vi "Color Pixel with Color Scale.vi"(6 "Color Scale 1D Color Array":T2(array[cluster]), 7 "Limit+NaN Colors":T1, 8 "Error In":errorcluster, 9 "Color Scale Min Value":sgl, 10 "Color Scale Max Value":sgl, 11 "Pixel Value":sgl) -> (0 "Error Out":errorcluster, 3 "Pixel Color":T3)   [LabVIEW 2021, in "Image.lvlib"]
uses:
  Palette/Limit+NaN Colors.ctl
  Image.lvlib
  Palette/Palette.lvlib
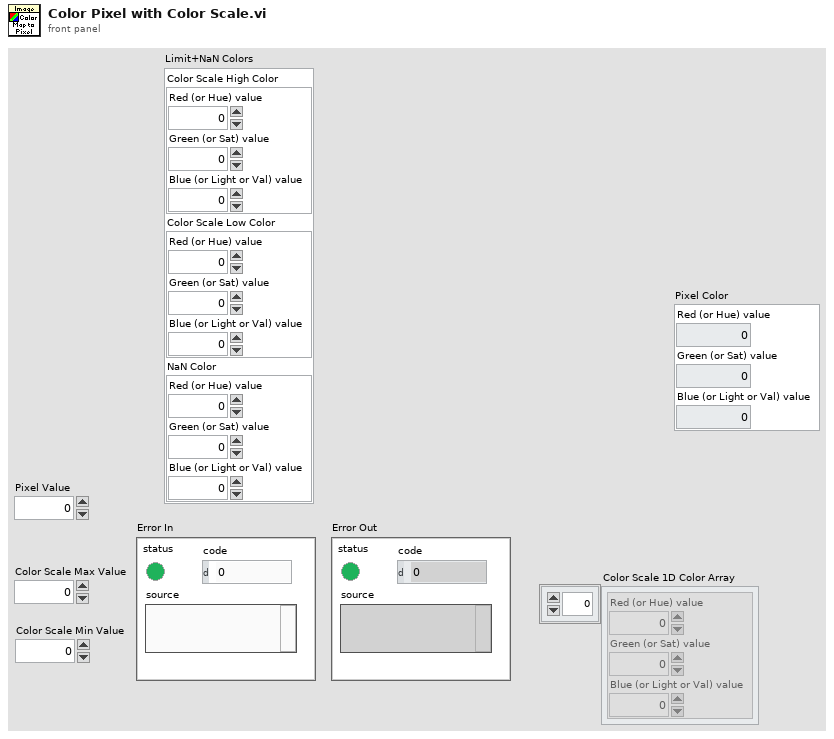
[diagram p1: front panel]
types:
  T1 = typedef "Palette.lvlib/Limit+NaN Colors.ctl" = cluster{"Color Scale High Color":cluster{"Red (or Hue) value":u8, "Green (or Sat) value":u8, "Blue (or Light or Val) value":u8}, "Color Scale Low Color":cluster{"Red (or Hue) value":u8, "Green (or Sat) value":u8, "Blue (or Light or Val) value":u8}, "NaN Color":cluster{"Red (or Hue) value":u8, "Green (or Sat) value":u8, "Blue (or Light or Val) value":u8}}
  T2 = cluster{"Red (or Hue) value":u8, "Green (or Sat) value":u8, "Blue (or Light or Val) value":u8}[]
  T3 = cluster{"Red (or Hue) value":u8, "Green (or Sat) value":u8, "Blue (or Light or Val) value":u8}
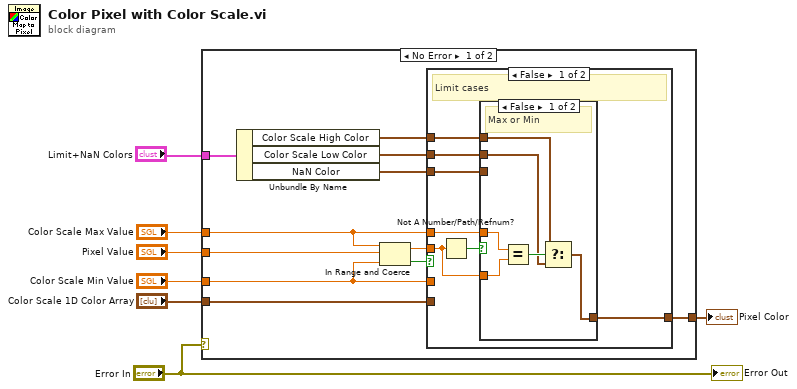
[diagram p0: block diagram]
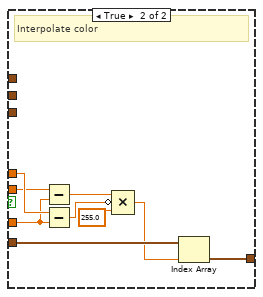
[diagram p3: hidden frame]
diagram:
  n1 = case shown="No Error" "Error In" {
    tunnel: [w17 _] -> w7
    tunnel: "Color Scale 1D Color Array" -> [w16 _]
    tunnel: "Color Scale Min Value" -> [w12 _]
    tunnel: "Color Scale Max Value" -> [w13 _]
    tunnel: "Pixel Value" -> [w14 _]
    tunnel: "Limit+NaN Colors" -> [w11 _]
    frame No Error {
      n2 = Unbundle By Name(w11) -> ("Color Scale High Color"=w9:T3, "Color Scale Low Color"=w8:T3, "NaN Color"=w10:T3)
      n3 = In Range and Coerce(upper limit=w13, x=w14, lower limit=w12) -> (coerced(x)=w15:sgl, In Range?=w18:bool)
      n4 = case shown="False" w18 {
        tunnel: w13 -> [w22 w41]
        tunnel: w15 -> [w23 w40]
        tunnel: w12 -> [_ w39]
        tunnel: w16 -> [_ w35]
        tunnel: [w24 w33] -> w17
        tunnel: w10 -> [w21 _]
        tunnel: w9 -> [w20 _]
        tunnel: w8 -> [w19 _]
        frame False {
          # "Limit cases"
          n5 = Not A Number/Path/Refnum?(number/path/refnum=w23) -> (NaN/Path/Refnum?=w25:bool)
          n6 = case shown="False" w25 {
            tunnel: [w30 w32] -> w24
            tunnel: w23 -> [w29 _]
            tunnel: w22 -> [w28 _]
            tunnel: w21 -> [_ w32]
            tunnel: w20 -> [w27 _]
            tunnel: w19 -> [w26 _]
            frame False {
              # "Max or Min"
              n7 = Equal?(x=w28, y=w29) -> (x = y?=w31:bool)
              n8 = Select(t=w27, s=w31, f=w26) -> (s? t:f=w30:T3)
            }
            frame True {
              # "NaN"
            }
          }
        }
        frame True {
          # "Interpolate color"
          n9 = Subtract(x=w40, y=w39) -> (x-y=w38:sgl)
          n10 = Subtract(x=w41, y=w39) -> (x-y=w37:sgl)
          n11 = Compound Arithmetic op=MULTIPLY(w38, invert w37, sgl 255.0 ("value")) -> (w34:sgl)
          n12 = Index Array(array=w35, index=w34) -> (element=w33:T3)
        }
      }
    }
    frame Error {
    }
  }
  "Pixel Color" <- w7
  "Error Out" <- "Error In"
